vi "IsErrorCluster.vi"(8 "error in (no error)":errorcluster, 11 "cluster elements info":variant[](array[variant])) -> (0 "error out":errorcluster, 3 "IsErrClust?":bool)   [LabVIEW 2019, in "BlueVariantView.lvlib"]
uses:
  BlueVariantView.lvlib
  <vilib>/Utility/Data Type/Type Definitions/Data Type.ctl
  <vilib>/Utility/Data Type/NI_Data Type.lvlib
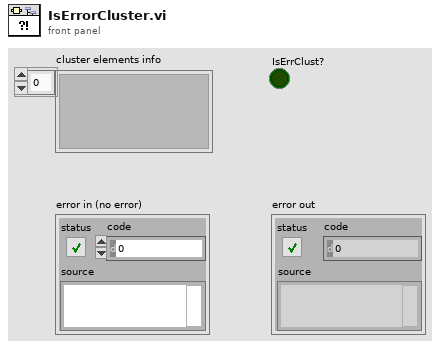
[diagram p1: front panel]
types:
  T1 = typedef "NI_Data Type.lvlib/Data Type.ctl" = enum8{"Invalid Type", "Void", "I8", "I16", "I32", "I64", "U8", "U16", "U32", "U64", "Single Float", "Double Float", "Extended Float", "Single Complex", "Double Complex", "Extended Complex", "Enum U8", "Enum U16", "Enum U32", "Enum U64", "Single Float With Unit", "Double Float With Unit", "Extended Float With Unit", "Single Complex with Unit", "Double Complex with Unit", "Extended Complex with Unit", "Boolean", "String", "Path", "Picture", "Tag", "Array", "Cluster", "Variant", "LV Variant", "Waveform", "Timestamp", "Digital Waveform", "Digital Data", "ExpressData", "Refnum", "External Data", "VI", "Poly VI", "LabVIEW Class Instance", "Fixed Point", "Set Collection", "Map Collection"}
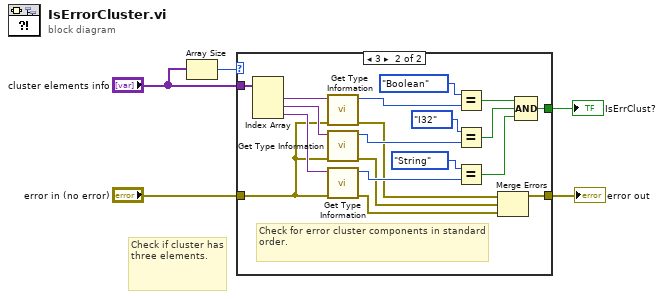
[diagram p0: block diagram]
diagram:
  # "Check if cluster has three elements."
  n1 = Array Size(array="cluster elements info") -> (size(s)=w5:i32)
  n2 = case shown="3" w5 {
    tunnel: "cluster elements info" -> [_ w25]
    tunnel: [_ w21] -> w3
    tunnel: "error in (no error)" -> [w6 w13]
    tunnel: [w6 w20] -> w1
    frame Default {
      # "Cluster does not have the right number of elements."
    }
    frame 3 {
      # "Check for error cluster components in standard order."
      n3 = Index Array(array=w25) -> (element #1=w11:variant, element #2=w14:variant, element #3=w15:variant)  [unwired: 3 in]
      n4 = call <vilib>:"Get Type Information.vi"("error in (no error)"=w13, "variant"=w11) -> ("error out"=w12:errorcluster, "type"=w10:T1)  [unwired: 5 in, 3 out]
      n5 = call <vilib>:"Get Type Information.vi"("error in (no error)"=w13, "variant"=w14) -> ("error out"=w17:errorcluster, "type"=w16:T1)  [unwired: 5 in, 3 out]
      n6 = call <vilib>:"Get Type Information.vi"("error in (no error)"=w13, "variant"=w15) -> ("error out"=w19:errorcluster, "type"=w18:T1)  [unwired: 5 in, 3 out]
      n7 = Equal?(x=Data_Type."Boolean" ("Type"), y=w10) -> (x = y?=w24:bool)
      n8 = Equal?(x=Data_Type."I32" ("Type"), y=w16) -> (x = y?=w23:bool)
      n9 = Equal?(x=Data_Type."String" ("Type"), y=w18) -> (x = y?=w22:bool)
      n10 = Merge Errors(w12, w17, w19) -> (w20:errorcluster)
      n11 = Compound Arithmetic op=AND(w24, w23, w22) -> (w21:bool)
    }
  }
  "error out" <- w1
  "IsErrClust?" <- w3
